vi "decay_analysis.vi"() -> ()   [LabVIEW 2014]
uses:
  <vilib>/gmath/SpecialFunctions.llb/Factorial.vi
  <vilib>/Utility/file.llb/Read From Spreadsheet File (DBL).vi
  <vilib>/imath/engines/lvmath2/RunTimeEngine/Managers/WorkSpace/UID Generator.vi
  <vilib>/imath/engines/lvmath2/RunTimeEngine/BuiltInFunctions/sum/NIMS_sum(GV).vi
  <instcachedir>/0/NIMS_sum(GV)_67F5EC36BC034E54A6BEC5B0673C00E5.lvgen/NIMS_sum(GV)_67F5EC36BC034E54A6BEC5B0673C00E5_000.vi
  <vilib>/imath/engines/lvmath2/RunTimeEngine/IndexRead/NIMS V(S).vi
  <instcachedir>/0/NIMS V(S)_0488751826AF41519A22953C041130DC.lvgen/NIMS V(S)_0488751826AF41519A22953C041130DC_000.vi
  <vilib>/imath/engines/lvmath2/RunTimeEngine/RunTimeType/NIMS_RunTimeType_From StrictType (excl LVString).vi
  <instcachedir>/0/NIMS_RunTimeType_From StrictType (excl LVString)_6F30FCEAD152B34FB6BC3D48AAFE00E6.lvgen/NIMS_RunTimeType_From StrictType (excl LVString)_6F30FCEAD152B34FB6BC3D48AAFE00E6_000.vi
  <vilib>/imath/engines/lvmath2/RunTimeEngine/ErrorHandling/NIMS_Create Error From Enums.vi
  <vilib>/imath/engines/lvmath2/RunTimeEngine/LocalVariableDefStatement/MC_LocalVariableDefStatement_Display.vi
  <vilib>/imath/engines/lvmath2/RunTimeEngine/BuiltInFunctions/length/NIMS_length(GV).vi
  <instcachedir>/0/NIMS_length(GV)_08A3D13377FD4E4B96F5795FBF3698FA.lvgen/NIMS_length(GV)_08A3D13377FD4E4B96F5795FBF3698FA_000.vi
  <vilib>/imath/engines/lvmath2/RunTimeEngine/BuiltInFunctions/zeros/NIMS_V=zeros(I32,I32).vi
  <vilib>/imathl/engines/lvmath/Functions/Error Handling/Create Error.vi
  <vilib>/imath/engines/lvmath2/RunTimeEngine/RangeToken/NIMS_Range_R2 - Integer.vi
  <instcachedir>/0/NIMS_Range_R2 - Integer_F15DFB86DF44D24783EFA65F7BB7CC2E.lvgen/NIMS_Range_R2 - Integer_F15DFB86DF44D24783EFA65F7BB7CC2E_000.vi
  <vilib>/imath/engines/lvmath2/RunTimeEngine/CommandStatement/MC_CommandStatement_break.vi
  <vilib>/imath/engines/lvmath2/RunTimeEngine/ArithmeticOperatorToken/NIMS_ArithmeticOperator_power(S).vi
  <instcachedir>/0/NIMS_ArithmeticOperator_power(S)_7E7603DDFF3F9240B7D001B368291B9B.lvgen/NIMS_ArithmeticOperator_power(S)_7E7603DDFF3F9240B7D001B368291B9B_014.vi
  <vilib>/imath/engines/lvmath2/RunTimeEngine/IndexReplace/NIMS V(S)=S.vi
  <instcachedir>/0/NIMS V(S)=S_EEB296E3296AB441BB925DBFA05F08B2.lvgen/NIMS V(S)=S_EEB296E3296AB441BB925DBFA05F08B2_001.vi
  <vilib>/imath/engines/lvmath2/RunTimeEngine/Managers/SymbolTable/Clear UID.vi
  <vilib>/imath/engines/lvmath2/RunTimeEngine/NodeEndStatement/NIMS_NodeEndStatement_Output.vi
  <instcachedir>/0/NIMS_NodeEndStatement_Output_53EC0D466D134D7ABD903AC30B43404B.lvgen/NIMS_NodeEndStatement_Output_53EC0D466D134D7ABD903AC30B43404B_005.vi
  <instcachedir>/0/NIMS_NodeEndStatement_Output_53EC0D466D134D7ABD903AC30B43404B.lvgen/NIMS_NodeEndStatement_Output_53EC0D466D134D7ABD903AC30B43404B_000.vi
  <vilib>/imath/engines/lvmath2/RunTimeEngine/ErrorHandling/NIMS_Finalize Error.vi
  <vilib>/gmath/NI_Gmath.lvlib
  <vilib>/imath/engines/lvmath2/RunTimeEngine/Managers/SymbolTable/NIMS_WorkSpace.lvlib
panel:
  out "Constant Rate":cluster{"pspan":dbl[], "pdist":dbl[]}[](graph)=[{"pspan"=[0.0, 1.0, 2.0], "pdist"=[984.0, 197.0, 0.0]}, {"pspan"=[0.0, 0.01, 0.02, 0.03, 0.04, 0.05, 0.06, 0.07, 0.08, 0.09, 0.1, 0.11, 0.12, 0.13, 0.14, 0.15, 0.16, 0.17, 0.18, 0.19, 0.2, 0.21, 0.22, 0.23, 0.24, 0.25, 0.26, 0.27, 0.28, 0.29, 0.3, 0.31, 0.32, 0.33, 0.34, 0.35000000000000003, 0.36, 0.37, 0.38, 0.39, 0.4, 0.41000000000000003, 0.42, 0.43, 0.44, 0.45, 0.46, 0.47000000000000003, 0.48, 0.49, 0.5, 0.51, 0.52, 0.53, 0.54, 0.55, 0.56, 0.5700000000000001, 0.58, 0.59, 0.6, 0.61, 0.62, 0.63, 0.64, 0.65, 0.66, 0.67, 0.68, 0.6900000000000001, 0.7000000000000001, 0.71, 0.72, 0.73, 0.74, 0.75, 0.76, 0.77, 0.78, 0.79, 0.8, 0.81, 0.8200000000000001, 0.8300000000000001, 0.84, 0.85, 0.86, 0.87, 0.88, 0.89, 0.9, 0.91, 0.92, 0.93, 0.9400000000000001, 0.9500000000000001, 0.96, 0.97, 0.98, 0.99, 1.0, 1.01, 1.02, 1.03, 1.04, 1.05, 1.06, 1.07, 1.08, 1.09, 1.1, 1.11, 1.12, 1.1300000000000001, 1.1400000000000001, 1.1500000000000001, 1.16, 1.17, 1.18, 1.19, 1.2, 1.21, 1.22, 1.23, 1.24, 1.25, 1.26, 1.27, 1.28, 1.29, 1.3, 1.31, 1.32, 1.33, 1.34, 1.35, 1.36, 1.37, 1.3800000000000001, 1.3900000000000001, 1.4000000000000001, 1.41, 1.42, 1.43, 1.44, 1.45, 1.46, 1.47, 1.48, 1.49, 1.5, 1.51, 1.52, 1.53, 1.54, 1.55, 1.56, 1.57, 1.58, 1.59, 1.6, 1.61, 1.62, 1.6300000000000001, 1.6400000000000001, 1.6500000000000001, 1.6600000000000001, 1.67, 1.68, 1.69, 1.7, 1.71, 1.72, 1.73, 1.74, 1.75, 1.76, 1.77, 1.78, 1.79, 1.8, 1.81, 1.82, 1.83, 1.84, 1.85, 1.86, 1.87, 1.8800000000000001, 1.8900000000000001, 1.9000000000000001, 1.9100000000000001, 1.92, 1.93, 1.94, 1.95, 1.96, 1.97, 1.98, 1.99, 2.0], "pdist"=[999.553846762726, 981.8120503831359, 964.3851658412566, 947.2676035415694, 930.4538731022864, 913.938581594334, 897.7164318115947, 881.7822205718531, 866.1308370478976, 850.7572611282447, 835.6565618069624, 820.8238956020701, 806.254505002015, 791.9437169397202, 777.8869412937197, 764.0796694158981, 750.517472685361, 737.1960010879741, 724.1109818211175, 711.2582179232012, 698.6335869275097, 686.2330395399381, 674.0525983402007, 662.0883565060893, 650.336476560379, 638.7931891399733, 627.4547917868983, 616.3176477607558, 605.3781848722547, 594.6328943374479, 584.0783296523041, 573.711105487259, 563.5278966013843, 553.525436775832, 543.7005177662093, 534.0499882735489, 524.5707529335434, 515.2597713237209, 506.11405698824314, 497.1306764800141, 488.3067484197883, 479.63944257198216, 471.12597893688877, 462.76362685900466, 454.5497041511848, 446.48157623434264, 438.5566552924211, 430.7723994423616, 423.1263119188067, 415.6159402732735, 408.23887558754205, 400.99275170100543, 393.8752444517341, 386.88407093101154, 380.0169887511014, 373.27179532601167, 366.6463271650251, 360.1384591787688, 353.7461039976019, 347.4672113021006, 341.2997671654274, 335.2417934073734, 329.29134695986534, 323.4465192437356, 317.7054355565536, 312.0662544713235, 306.5271672458547, 301.08639724261593, 295.7421993588866, 290.4928594670228, 285.3366938646585, 280.272048734666, 275.29729961470053, 270.41085087616204, 265.611135212404, 260.8966131360272, 256.2657724850954, 251.71712793811662, 247.24922053763274, 242.8606172222655, 238.54991036706807, 234.31571733203623, 230.15668001863233, 226.0714644341813, 222.0587602639986, 218.11728045111232, 214.24576078344586, 210.44295948832703, 206.70765683419552, 203.03865473937884, 199.4347763878136, 195.8948658515865, 192.41778772017594, 189.00242673627395, 185.64768743807247, 182.35249380789887, 179.115788927088, 175.93653463698033, 172.81371120593712, 169.74631700226612, 166.73336817295262, 163.77389832809294, 160.86695823092933, 158.01161549338624, 155.2069542770114, 152.4520749992242, 149.74609404477914, 147.08814348234975, 144.47737078614378, 141.91293856245912, 139.39402428109364, 136.91982001152226, 134.48953216375693, 132.10238123380597, 129.7576015536518, 127.45444104566633, 125.19216098138537, 122.97003574456473, 120.78735259844215, 118.6434114571301, 116.53752466106637, 114.4690167564503, 112.437224278594, 110.44149553911903, 108.48119041693026, 106.5556801528999, 104.66434714819559, 102.80658476618873, 100.98179713787825, 99.18939897076818, 97.42881536113796, 95.69948160964441, 94.00084304019704, 92.33235482204817, 90.69348179504085, 89.08369829795862, 87.50248799992212, 85.94934373477814, 84.42376733842835, 82.9252694890455, 81.45336955012553, 80.00759541632557, 78.58748336203818, 77.19257789265363, 75.82243159846185, 74.4766050111478, 73.15466646283403, 71.85619194762512, 70.58076498560959, 69.32797648927595, 34.04871231614979, 33.444357360329406, 32.85072953301931, 32.26763843074058, 31.694897029621917, 31.13232162541249, 30.57973177455967, 30.036950236332533, 29.503802915972727, 28.980118808854286, 28.465729945634713, 27.960471338379577, 27.464180927643305, 26.976699530489377, 26.49787078943313, 26.027541122290735, 25.565559672918443, 25.111778262826146, 24.666051343649738, 24.22823595046719, 23.798191655943164, 23.375780525287553, 22.96086707201355, 22.55331821448091, 22.153003233210665, 21.759793728957394, 21.373563581525747, 20.99418890931795, 20.62154802959935, 20.255521419469222, 19.895991677524304, 19.54284348620285, 19.195963574797027, 18.855240683121814, 18.520565525828843, 18.191830757353568, 17.868930937484684, 17.55176249754463, 17.240223707170408, 16.934214641684004, 16.633637150042023, 16.338394823354168, 16.048392963960485, 15.763538555057574, 15.483740230863798, 15.208908247314179, 14.938954453275334, 14.673792262271435, 14.413336624711945, 14.157504000612374, 13.906212332799182]}]
  in  "Path 2":path=path "/Macintosh HD/Users/barthamre/Documents/preShakeData"
  out "Decay  Plot":cluster{"all rows":dbl[], "all rows":dbl[]}[](graph)=[{"all rows"=[1.0, 2.0, 3.0, 4.0, 5.0, 6.0, 7.0, 8.0, 9.0, 10.0, 11.0, 12.0, 13.0, 14.0, 15.0, 16.0, 17.0, 18.0, 19.0, 20.0, 21.0, 22.0, 23.0, 24.0, 25.0, 26.0, 27.0, 28.0, 29.0, 30.0, 31.0, 32.0, 33.0, 34.0, 35.0, 36.0, 37.0, 38.0, 39.0, 40.0, 41.0, 42.0, 43.0, 44.0, 45.0, 46.0, 47.0, 48.0, 49.0, 50.0, 51.0, 52.0, 53.0, 54.0, 55.0, 56.0, 57.0, 58.0, 59.0, 60.0, 61.0, 62.0, 63.0, 64.0, 65.0, 66.0, 67.0, 68.0, 69.0, 70.0, 71.0, 72.0, 73.0, 74.0, 75.0, 76.0, 77.0, 78.0, 79.0, 80.0, 81.0, 82.0, 83.0, 84.0, 85.0, 86.0, 87.0, 88.0, 89.0, 90.0, 91.0, 92.0, 93.0, 94.0, 95.0, 96.0, 97.0, 98.0, 99.0, 100.0, 101.0, 102.0, 103.0, 104.0, 105.0, 106.0, 107.0, 108.0, 109.0, 110.0, 111.0, 112.0, 113.0, 114.0, 115.0, 116.0, 117.0, 118.0, 119.0, 120.0, 121.0, 122.0, 123.0, 124.0, 125.0, 126.0, 127.0, 128.0, 129.0, 130.0, 131.0, 132.0, 133.0, 134.0, 135.0, 136.0, 137.0, 138.0, 139.0, 140.0, 141.0, 142.0, 143.0, 144.0, 145.0, 146.0, 147.0, 148.0, 149.0, 150.0, 151.0, 152.0, 153.0, 154.0, 155.0, 156.0, 157.0, 158.0, 159.0, 160.0, 161.0, 162.0, 163.0, 164.0, 165.0, 166.0, 167.0, 168.0, 169.0, 170.0, 171.0, 172.0, 173.0, 174.0, 175.0, 176.0, 177.0, 178.0, 179.0, 180.0, 181.0, 182.0, 183.0, 184.0, 185.0, 186.0, 187.0, 188.0, 189.0, 190.0, 191.0, 192.0, 193.0, 194.0, 195.0, 196.0, 197.0, 198.0, 199.0, 200.0, 201.0, 202.0, 203.0, 204.0, 205.0, 206.0, 207.0, 208.0, 209.0, 210.0, 211.0, 212.0, 213.0, 214.0, 215.0, 216.0, 217.0, 218.0, 219.0, 220.0, 221.0, 222.0, 223.0, 224.0, 225.0, 226.0, 227.0, 228.0, 229.0, 230.0, 231.0, 232.0, 233.0, 234.0, 235.0, 236.0, 237.0, 238.0, 239.0, 240.0, 241.0, 242.0, 243.0, 244.0, 245.0, 246.0, 247.0, 248.0, 249.0, 250.0, 251.0, 252.0, 253.0, 254.0, 255.0, 256.0, 257.0, 258.0, 259.0, 260.0, 261.0, 262.0, 263.0, 264.0, 265.0, 266.0, 267.0, 268.0, 269.0, 270.0, 271.0, 272.0, 273.0, 274.0, 275.0, 276.0, 277.0, 278.0, 279.0, 280.0, 281.0, 282.0, 283.0, 284.0, 285.0, 286.0, 287.0, 288.0, 289.0, 290.0, 291.0, 292.0, 293.0, 294.0, 295.0, 296.0, 297.0, 298.0, 299.0, 300.0], "all rows"=[63.1786187295882, 62.637305733792985, 62.100625295975945, 61.56853777069426, 61.041003851790926, 60.517984569491105, 59.9994412875234, 59.48533570026572, 58.975629829915604, 58.47028602368468, 57.96926695101727, 57.47253560083266, 56.98005527879106, 56.49178960458297, 56.00770250924161, 55.52775823247856, 55.05192132004201, 54.58015662109773, 54.11242928563243, 53.648704761879294, 53.188948793765654, 52.73312741838237, 52.28120696347494, 51.833154044956174, 51.38893556443991, 50.94851870679611, 50.51187093772665, 50.07896000136206, 49.64975391787866, 49.22422098113619, 48.802329756335595, 48.384049077696936, 47.96934804615709, 47.55819602708718, 47.15056264802957, 46.74641779645421, 46.34573161753413, 45.948474511940056, 45.55461713365385, 45.16413038780066, 44.776985428499664, 44.39315365673316, 44.01260671823388, 43.63531650139049, 43.26125513517086, 42.89039498706325, 42.52270866103501, 42.15816899550881, 41.79674906135616, 41.43842215990814, 41.083161820983086, 40.73094180093121, 40.38173608069597, 40.03551886389196, 39.6922645748993, 39.351947856974334, 39.01454357037649, 38.68002679051115, 38.34837280608844, 38.01955711729777, 37.69355543399799, 37.37034367392304, 37.049897960902946, 36.73219462310007, 36.41721019126041, 36.10492139697989, 35.79530517098552, 35.488338641431184, 35.1839991322081, 34.88226416126965, 34.583111438970676, 34.28651886642081, 33.99246453385209, 33.700926719000364, 33.411883885500686, 33.12531468129637, 32.841197937061715, 32.55951266463812, 32.28023805548372, 32.0033534791362, 31.728838481688793, 31.456672784279316, 31.186836281592146, 30.919309040372987, 30.654071297956406, 30.39110346080589, 30.13038610306647, 29.871899965129696, 29.615625952210884, 29.36154513293857, 29.109638737956022, 28.8598881585347, 28.612274945199623, 28.366780806366446, 28.123387606990256, 27.88207736722591, 27.64283226109981, 27.405634615193083, 27.170466907336042, 26.937311765313748, 26.70615196558273, 26.47697043199865, 26.249750234554853, 26.024474588131717, 25.80112685125672, 25.579690524875108, 25.36014925113108, 25.14248681215939, 24.926687128887348, 24.712734259846986, 24.50061239999748, 24.290305879557565, 24.081799162848007, 23.875076847143976, 23.67012366153717, 23.466924465807775, 23.265464249306017, 23.06572812984328, 22.867701352592796, 22.671369288999603, 22.476717435699967, 22.28373141344997, 22.09239696606331, 21.902699959358156, 21.714626380113035, 21.528162335031663, 21.343294049716633, 21.16000786765185, 20.978290249193726, 20.798127770570964, 20.61950712289295, 20.442415111166596, 20.26683865332157, 20.092764779243957, 19.9201806298181, 19.749073455976678, 19.579430617758938, 19.41123958337693, 19.244487928289775, 19.079163334285855, 18.91525358857284, 18.75274658287549, 18.591630312541223, 18.431892875653325, 18.27352247215169, 18.116507402961158, 17.96083606912729, 17.80649697095953, 17.653478707181698, 17.501769974089772, 17.351359564716844, 17.202236368005266, 17.054389367985852, 16.9078076429641, 16.7624803647134, 16.618396797675135, 16.47554629816563, 16.333918313589862, 16.193502381661965, 16.054288129632333, 15.916265273521374, 15.779423617359829, 15.643753052435555, 15.509243556546805, 15.375885193261851, 15.243668111184984, 15.112582543228756, 14.982618805892475, 14.853767298546876, 14.726018502724912, 14.599362981418587, 14.473791378381852, 14.349294417439426, 14.225862901801573, 14.103487713384698, 13.982159812137787, 13.861870235374608, 13.742610097111621, 13.624370587411555, 13.507142971732605, 13.390918590283198, 13.275688857382267, 13.161445260825044, 13.048179361254219, 12.935882791536526, 12.824547256144644, 12.714164530544402, 12.604726460587207, 12.496224961907691, 12.388652019326505, 12.281999686258231, 12.176260084124342, 12.071425401771208, 11.967487894893072, 11.86443988545996, 11.76227376115051, 11.660981974789616, 11.560557043790912, 11.460991549604033, 11.362278137166589, 11.26440951436082, 11.167378451474939, 11.071177780669046, 10.975800395445635, 10.881239250124622, 10.78748735932287, 10.69453779743817, 10.602383698137638, 10.511018253850475, 10.420434715265095, 10.330626390830542, 10.241586646262158, 10.153308904051524, 10.065786642980546, 9.979013397639731, 9.892982757950577, 9.807688368692055, 9.723123929031129, 9.639283192057304, 9.556159964321168, 9.473748105376867, 9.392041527328484, 9.311034194380348, 9.230720122391128, 9.151093378431796, 9.072148080347349, 8.993878396322275, 8.916278544449758, 8.839342792304551, 8.76306545651952, 8.6874409023658, 8.612463543336553, 8.538127840734273, 8.464428303261647, 8.391359486615892, 8.318915993086598, 8.247092471156957, 8.175883615108463, 8.105284164628959, 8.035288904424052, 7.965892663831859, 7.897090316441026, 7.828876779712044, 7.761247014601786, 7.694196025191279, 7.627718858316628, 7.561810603203127, 7.496466391102496, 7.4316813949332134, 7.367450828923934, 7.303769948259954, 7.240634048732705, 7.178038466392256, 7.115978577202761, 7.054449796700889, 6.993447579657156, 6.932967419740163, 6.87300484918371, 6.813555438456747, 6.754614795936165, 6.696178567582372, 6.638242436617667, 6.580802123207334, 6.523853384143499, 6.4673920125316675, 6.4114138374799605, 6.355914723791004, 6.30089057165645, 6.24633731635412, 6.1922509279477485, 6.138627410989261, 6.085462804223646, 6.032753180296316, 5.980494645463002, 5.9286833393021015, 5.877315434429513, 5.826387136215897, 5.775894682506358, 5.725834343342541, 5.676202420687075, 5.626995248150407, 5.5782091907199485, 5.529840644491566, 5.481886036403343, 5.434341823971635, 5.38720449502938, 5.3404705674666575, 5.294136588973445, 5.248199136784602, 5.202654817427018, 5.157500266468937, 5.112732148271415, 5.068347155741917, 5.024342010090013, 4.980713460585168, 4.937458284316614, 4.8945732859552535, 4.852055297517627, 4.809901178131885, 4.768107813805767]}, ...(2 in all)]
  in  "Path":path=path "/Macintosh HD/Users/barthamre/Documents/decayData"
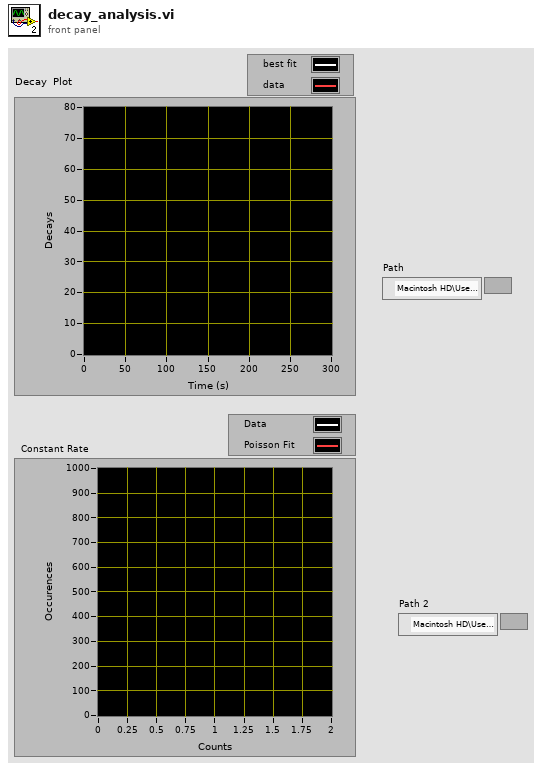
[diagram p1: front panel]
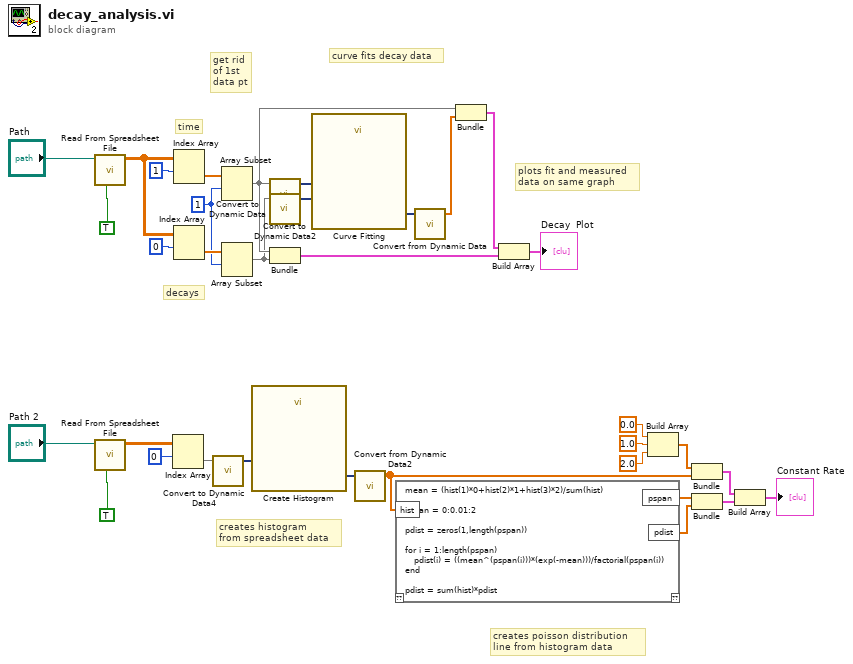
[diagram p0: block diagram]
diagram:
  w19 = 1 ("index")
  # "creates poisson distribution\nline from histogram data"
  # "creates histogram\nfrom spreadsheet data"
  # "plots fit and measured\ndata on same graph"
  # "curve fits decay data"
  # "get rid\nof 1st\ndata pt"
  # "decays"
  # "time"
  n1 = call-poly <vilib>:"Read From Spreadsheet File.vi"("transpose (no:F)"=TRUE, "file path (dialog if empty)"="Path") -> ("all rows"=w30:dbl[][])  [unwired: 5 in, 4 out]
  n2 = call-poly <vilib>:"Read From Spreadsheet File.vi"("transpose (no:F)"=TRUE, "file path (dialog if empty)"="Path 2") -> ("all rows"=w15:dbl[][])  [unwired: 5 in, 4 out]
  n3 = Index Array(array=w15, index (row)=0) -> (element=w12:dbl[])  [unwired: 1 in]
  n4 = Index Array(array=w30, index (row)=1 ("index")) -> (element=w21:dbl[])  [unwired: 1 in]
  n5 = Index Array(array=w30, index (row)=0 ("index")) -> (element=w20:dbl[])  [unwired: 1 in]
  n6 = call "Convert to Dynamic Data4"("Array"=w12) -> ("Dynamic Data Type"=w16:dynamicdata)  [unwired: 3 in]
  n7 = Array Subset(array=w21, index=w19) -> (w22:dbl[])  [unwired: 1 in]
  n8 = Array Subset(array=w20, index=w19) -> (w17:dbl[])  [unwired: 1 in]
  n9 = call "Create Histogram"("Signal"=w16) -> ("Histogram"=w11:dynamicdata)  [unwired: 9 in, 1 out]
  n10 = call "Convert to Dynamic Data2"("Array"=w22) -> ("Dynamic Data Type"=w29:dynamicdata)  [unwired: 3 in]
  n11 = call "Convert to Dynamic Data"("Array"=w17) -> ("Dynamic Data Type"=w31:dynamicdata)  [unwired: 3 in]
  n12 = Bundle(w22, w17) -> (w24:cluster{dbl[], dbl[]})  [unwired: 1 in]
  n13 = call "Curve Fitting"("Locations"=w29, "Signals"=w31) -> ("best fit"=w27:dynamicdata)  [unwired: 5 in, 4 out]
  n14 = call "Convert from Dynamic Data2"("Dynamic Data Type"=w11) -> ("Array"=w6:dbl[])  [unwired: 3 in]
  n15 = mathscript code="mean = (hist(1)*0+hist(2)*1+hist(3)*2)/sum(hist)\n\npspan = 0:0.01:2\n\npdist = zeros(1,length(pspan))\n\nfor i = 1:length(pspan)\n   pdist(i) = ((mean^(pspan(i)))*(exp(-mean)))/factorial(pspan(i))\nend\n\npdist = sum(hist)*pdist"("hist"=w6) -> ("pdist"=w4:cdb[], "pspan"=w5:dbl[])  [unwired: 1 in, 1 out]
  n16 = call "Convert from Dynamic Data"("Dynamic Data Type"=w27) -> ("Array"=w26:dbl[])  [unwired: 3 in]
  n17 = Bundle(w22, "Array"=w26) -> (w25:cluster{dbl[], "Array":dbl[]})  [unwired: 1 in]
  n18 = Build Array(w25, w24) -> (→"Decay  Plot":cluster{dbl[], "Array":dbl[]}[])
  n19 = Build Array(0.0 ("element"), 1.0 ("element"), 2.0 ("element")) -> (w7:dbl[])
  n20 = Bundle(w7, "Array"=w6) -> (w3:cluster{dbl[], "Array":dbl[]})  [unwired: 1 in]
  n21 = Bundle("pspan"=w5, "pdist"=w4) -> (w2:cluster{"pspan":dbl[], "pdist":cdb[]})  [unwired: 1 in]
  n22 = Build Array(w3, w2) -> (→"Constant Rate":cluster{"pspan":dbl[], "pdist":cdb[]}[])
